vi "TCP Check Connection.vi"(8 "error in (no error)":errorcluster, 11 "Connection In":T1) -> (0 "error out":errorcluster, 2 "Disconnected":bool, 3 "Connection out":T1)   [LabVIEW 2013]
doc: "This VI removes the host connection from the connection manager list if it becomes disconnected for any reason."
uses:
  stm_TCP Connection Info.ctl
  stm_MetaDataElement.ctl
  Connection Manager/TCP/TCP Connection Manager.vi
  NI STM.lvlib
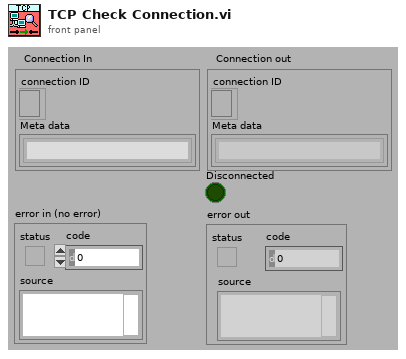
[diagram p1: front panel]
types:
  T1 = typedef "stm_TCP Connection Info.ctl" = cluster{"connection ID":refnum<k5>, "Meta data":T2[]}
  T2 = typedef "stm_MetaDataElement.ctl" = string
  T3 = typedef "NI STM.lvlib/TCP Connection Info.ctl" = cluster{"connection ID":refnum<k5>, "meta data":T4[]}
  T4 = typedef "NI STM.lvlib/MetaDataElement.ctl" = string
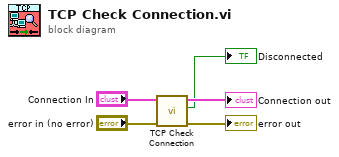
[diagram p0: block diagram]
diagram:
  n1 = call "TCP Check Connection.vi"("error in"="error in (no error)", "connection in"="Connection In") -> ("error out"=→"error out":errorcluster, "disconnected?"=→"Disconnected":bool, "connection out"=→"Connection out":T3)  [unwired: 7 in]
